vi "Sequence.Compile.vi"(8 "error in (no error)":errorcluster, 11 "State Variables":T10={"Aliases.All"=[], "Aliases.Outputs"=[], "UI.Sequence#ofColumns"=0, "SysDef.Path"=path "", "UI.SequenceRef"=refnum, "UI.StepInformationRef"=refnum, "UI.AbortRef"=refnum, "UI.GraphRef"=refnum, "UI.ViewRef"=refnum, "UI.IterationsRef"=refnum, "UI.IterationInformationRef"=refnum, "INI.Settings"={"Build Location"=path "C:/Simple Sequence Editor/SequenceRepo", "LoggingLocation"=path ""}}) -> (0 "error out":errorcluster, 1 "Warnings":string[](array[string]), 2 "CompiledSettings":T1)   [LabVIEW 2013, in "Simple Sequence Tools - Editor.lvlib"]
uses:
  Simple Sequence Tools - Editor.lvlib
  Types/StateVariables.ctl
  Shared/Types/ChannelProperties.ctl
  Shared/Types/INI.Settings
  Types/Compiled.RTSequenceProperties.ctl
  Types/Compiled.StepProperties.ctl
  Types/Compiled.IOStateProperties.ctl
  Types/Compiled.StepElementProperties.ctl
  Shared/Types/StepTypes.ctl
  Types/Compiled.StepCondition.ctl
  Types/OperationTypes.ctl
  Types/Compiled.SequenceChannels.ctl
  Shared/Simple Sequence Tools - Shared.lvlib
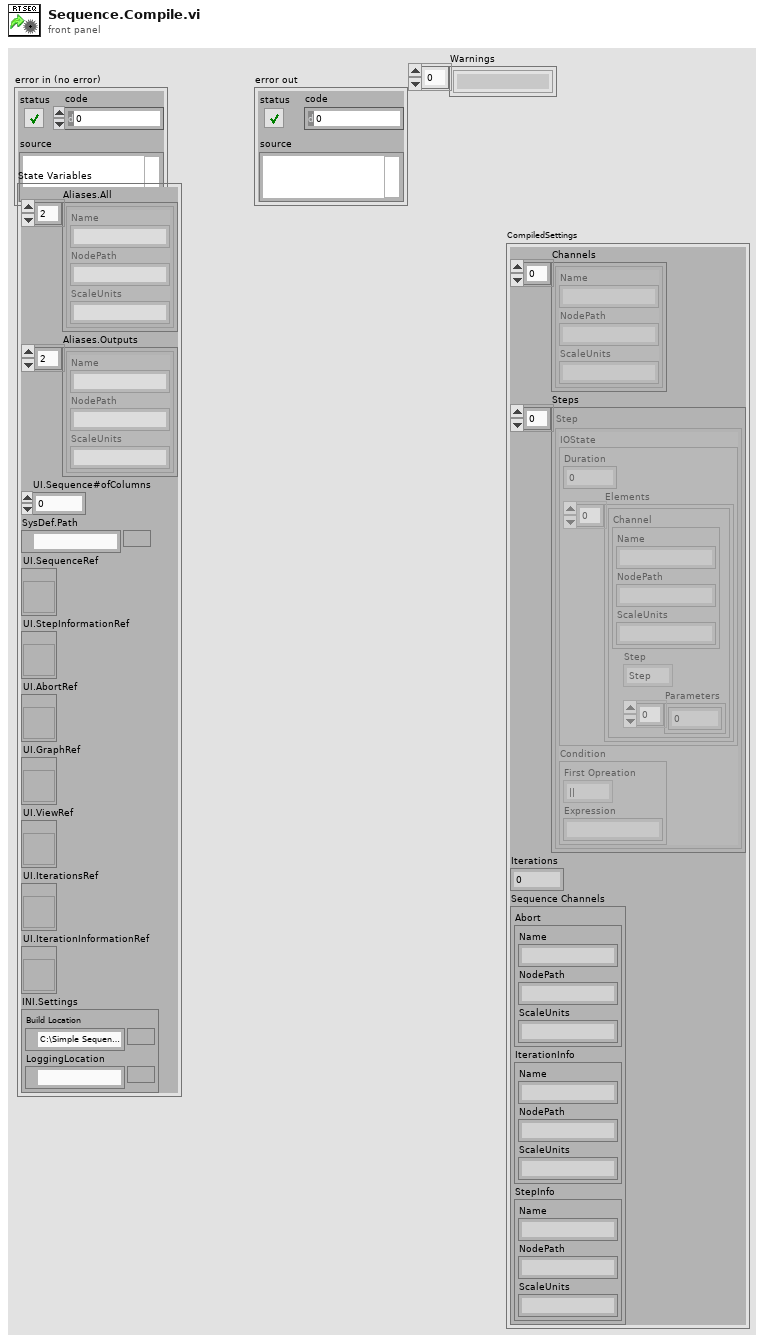
[diagram p1: front panel]
types:
  T1 = typedef "Simple Sequence Tools - Editor.lvlib/Compiled.RTSequenceProperties.ctl" = cluster{"Channels":T2[], "Steps":T3[], "Iterations":u32, "Sequence Channels":T9}
  T2 = typedef "Simple Sequence Tools - Shared.lvlib/ChannelProperties.ctl" = cluster{"Name":string, "NodePath":string, "ScaleUnits":string}
  T3 = typedef "Simple Sequence Tools - Editor.lvlib/Compiled.StepProperties.ctl" = cluster{"IOState":T4, "Condition":T7}
  T4 = typedef "Simple Sequence Tools - Editor.lvlib/Compiled.IOStateProperties.ctl" = cluster{"Duration":dbl, "Elements":T5[]}
  T5 = typedef "Simple Sequence Tools - Editor.lvlib/Compiled.StepElementProperties.ctl" = cluster{"Channel":T2, "Step":T6, "Parameters":dbl[]}
  T6 = typedef "Simple Sequence Tools - Shared.lvlib/StepTypes.ctl" = enum8{"Step", "iStep", "Ramp", "Unchanged", "Unknown"}
  T7 = typedef "Simple Sequence Tools - Editor.lvlib/Compiled.StepCondition.ctl" = cluster{"First Opreation":T8, "Expression":string}
  T8 = typedef "Simple Sequence Tools - Editor.lvlib/OperationTypes.ctl" = enum8{"None", "&&", "||"}
  T9 = typedef "Simple Sequence Tools - Editor.lvlib/Compiled.SequenceChannels.ctl" = cluster{"Abort":T2, "IterationInfo":T2, "StepInfo":T2}
  T10 = typedef "Simple Sequence Tools - Editor.lvlib/StateVariables.ctl" = cluster{"Aliases.All":T2[], "Aliases.Outputs":T2[], "UI.Sequence#ofColumns":i32, "SysDef.Path":path, "UI.SequenceRef":refnum<vi>, "UI.StepInformationRef":refnum<vi>, "UI.AbortRef":refnum<vi>, "UI.GraphRef":refnum<vi>, "UI.ViewRef":refnum<vi>, "UI.IterationsRef":refnum<vi>, "UI.IterationInformationRef":refnum<vi>, "INI.Settings":T11}
  T11 = typedef "Simple Sequence Tools - Shared.lvlib/INI.Settings" = cluster{"Build Location":path, "LoggingLocation":path}
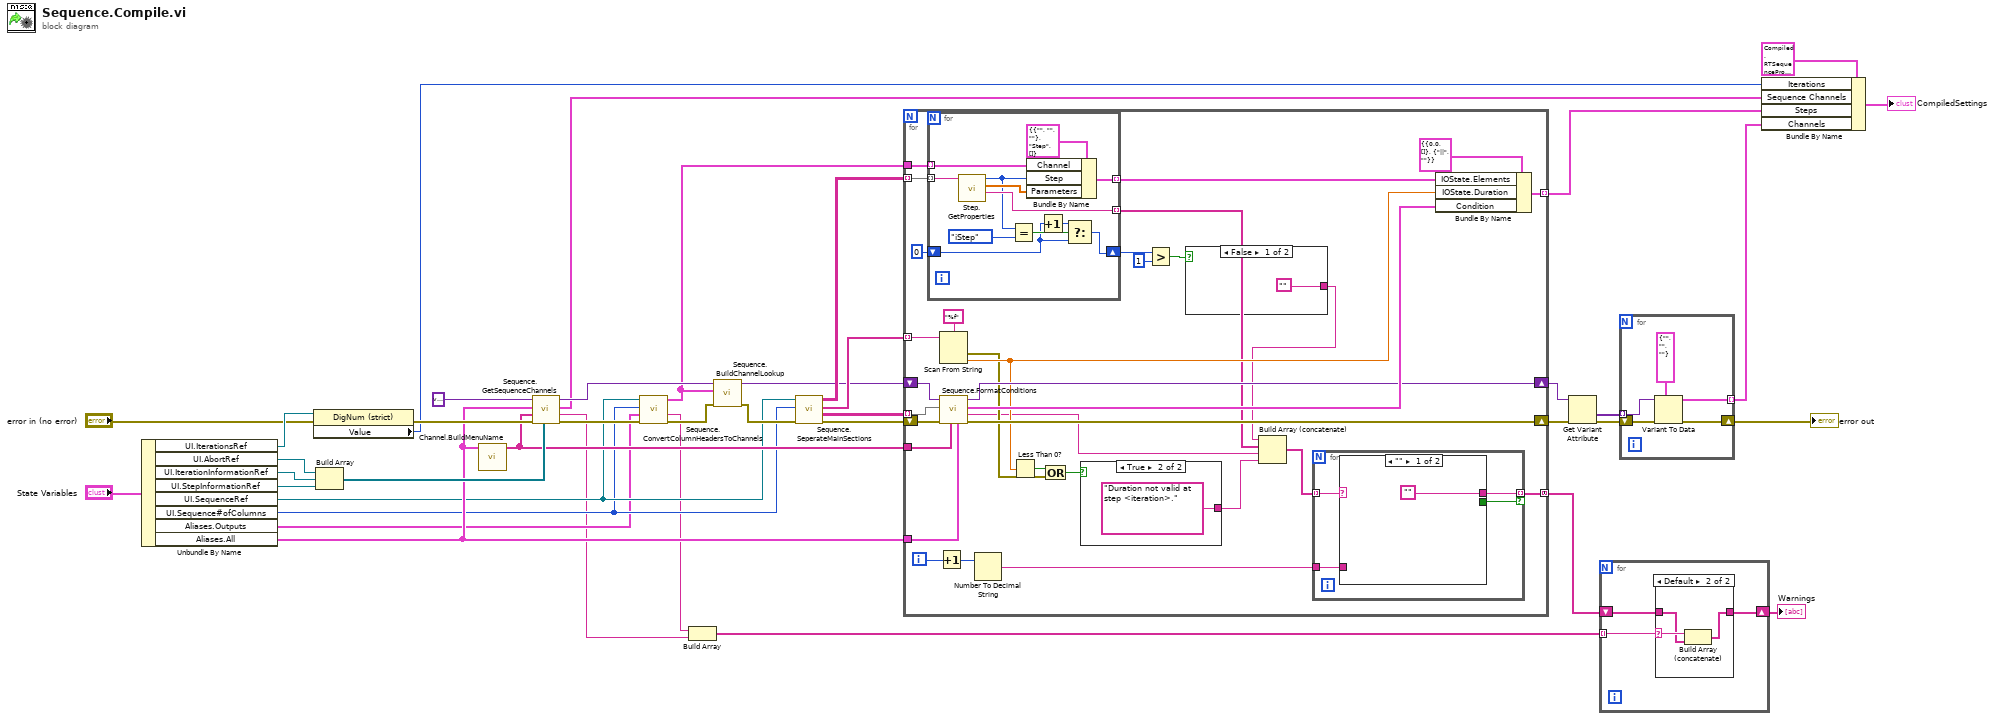
[diagram p0: block diagram]
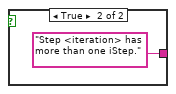
[diagram p3: hidden frame]
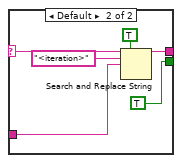
[diagram p4: hidden frame]
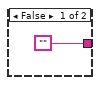
[diagram p5: hidden frame]
diagram:
  n1 = Unbundle By Name("State Variables") -> ("UI.IterationsRef"=w31:refnum<vi>, "UI.AbortRef"=w27:refnum<vi>, "UI.IterationInformationRef"=w26:refnum<vi>, "UI.StepInformationRef"=w25:refnum<vi>, "UI.SequenceRef"=w8:refnum<vi>, "UI.Sequence#ofColumns"=w7:i32, "Aliases.Outputs"=w6:T2[], "Aliases.All"=w20:T2[])
  n2 = property class="DigNum (strict)"(reference=w31, error in="error in (no error)") -> (error out=w24:errorcluster, "Value"=w12:u32)  [unwired: 1 out]
  n3 = Build Array(w27, w26, w25) -> (w23:refnum<vi>[])
  n4 = call "Channel.BuildMenuName.vi"("Aliases"=w20) -> ("Aliases Array"=w19:string[])  [unwired: 10 in]
  n5 = call "Sequence.GetSequenceChannels.vi"("Refs"=w23, "error in (no error)"=w24, "Aliases Array"=w19, "Aliases.All"=w20, "ChannelsLookup"=variant ("variant")) -> ("error out"=w10:errorcluster, "Warnings"=w4:string, "SequenceChannels"=w21:T9, "ChannelsLookup"=w22:variant)  [unwired: 3 in]
  n6 = call "Sequence.ConvertColumnHeadersToChannels.vi"("error in (no error)"=w10, "Aliases.Outputs"=w6, "UI.Sequence#ofColumns"=w7, "UI.SequenceRef"=w8) -> ("error out"=w9:errorcluster, "Warning"=w5:string, "Output Channels"=w16:T2[])  [unwired: 5 in]
  n7 = Build Array(w5, w4) -> (w3:string[])
  n8 = call "Sequence.BuildChannelLookup.vi"("error in (no error)"=w9, "Output Channels"=w16, "ChannelLookup"=w22) -> ("error out"=w18:errorcluster, "ChannelLookup"=w15:variant)  [unwired: 7 in]
  n9 = call "Sequence.SeperateMainSections.vi"("error in (no error)"=w18, "UI.Sequence#ofColumns"=w7, "MulticolumnListbox in"=w8) -> ("error out"=w17:errorcluster, "Conditions"=w36:string[][], "Duration"=w40:string[], "Steps"=w39:string[][])  [unwired: 5 in]
  n10 = for {
    tunnel: w40 -> [w72] mode=indexing
    tunnel: w39 -> [w71] mode=indexing
    tunnel: w16 -> [w70]
    tunnel: [w67] -> w14 mode=indexing
    tunnel: w36 -> [w62] mode=indexing
    tunnel: w19 -> [w63]
    tunnel: w20 -> [w64]
    shift-right: [w66] -> w29
    shift-left: w17 -> [w69]
    shift-right: [w59] -> w28
    shift-left: w15 -> [w61]
    tunnel: [w46] -> w2 mode=concatenating
    i -> [w49]
    n11 = for {
      tunnel: w71 -> [w99] mode=indexing
      tunnel: w70 -> [w97] mode=indexing
      tunnel: [w95] -> w65 mode=indexing
      tunnel: [w94] -> w51 mode=indexing
      shift-right: [w90] -> w44
      shift-left: 0 -> [w89]
      n12 = call "Step.GetProperties.vi"("String in"=w99) -> ("Warning"=w94:string, "Parameters"=w96:dbl[], "Step"=w93:T6)  [unwired: 8 in]
      n13 = Equal?(x=w93, y=StepTypes."iStep") -> (x = y?=w91:bool)
      n14 = Bundle By Name(cluster=T5 {"Channel"={"Name"="", "NodePath"="", "ScaleUnits"=""}, "Step"=enum."Step", "Parameters"=[]}, "Channel"=w97, "Step"=w93, "Parameters"=w96) -> (w95:T5)
      n15 = Increment(x=w89) -> (x+1=w88:i32)
      n16 = Select(t=w88, s=w91, f=w89) -> (s? t:f=w90:i32)
    }
    n17 = Increment(x=w49) -> (x+1=w48:i32)
    n18 = Scan From String(format string="%f", input string=w72) -> (error out=w55:errorcluster, output 1=w57:dbl)  [unwired: 3 in, 2 out]
    n19 = call "Sequence.FormatConditions.vi"("Aliases.All"=w64, "Aliases Array"=w63, "error in (no error)"=w69, "Conditions"=w62, "variant in"=w61) -> ("error out"=w66:errorcluster, "Warning"=w52:string, "Condition"=w60:T7, "variant out"=w59:variant)  [unwired: 3 in]
    n20 = Number To Decimal String(number=w48) -> (decimal integer string=w47:string)  [unwired: 1 in]
    n21 = Less Than 0?(x=w57) -> (x < 0?=w56:bool)
    n22 = Compound Arithmetic op=OR(w56, w55) -> (w54:bool)
    n23 = case shown="True" w54 {
      tunnel: ["" "Duration not valid at step <iteration>."] -> w53
      frame False {
      }
      frame True {
      }
    }
    n24 = Greater?(x=w44, y=1) -> (0:w42:bool)
    n25 = case shown="False" w42 {
      tunnel: ["" "Step <iteration> has more than one iStep."] -> w41
      frame False {
      }
      frame True {
      }
    }
    n26 = Build Array (concatenate)(w41, w51, w52, w53) -> (w50:string[])
    n27 = for {
      tunnel: w50 -> [w77] mode=indexing
      tunnel: w47 -> [w78]
      tunnel: [w76] -> w46 mode=indexing if=w75
      n28 = case shown="\"\"" w77 {
        selector: w77 -> [_ w82]
        tunnel: w78 -> [_ w83]
        tunnel: ["" w81] -> w76
        tunnel: [_ TRUE] -> w75
        frame "" {
        }
        frame Default {
          n29 = Search and Replace String(replace all?=TRUE ("replace all? (F)"), input string=w82, search string="<iteration>", replace string=w83) -> (result string=w81:string)  [unwired: 4 in, 3 out]
        }
      }
    }
    n30 = Bundle By Name(cluster=T3 {"IOState"={"Duration"=0.0, "Elements"=[]}, "Condition"={"First Opreation"=enum."||", "Expression"=""}} ("Step"), "IOState.Elements"=w65, "IOState.Duration"=w57, "Condition"=w60) -> (w67:T3)
  }
  n31 = Get Variant Attribute(Variant=w28, error in=w29) -> (values=w34:variant[], error out=w33:errorcluster)  [unwired: 2 in, 2 out]
  n32 = for {
    tunnel: w3 -> [w102] mode=indexing
    shift-right: [w100] -> w1
    shift-left: w2 -> [w101]
    n33 = case shown="Default" w102 {
      selector: w102 -> [_ w106]
      tunnel: w101 -> [w103 w105]
      tunnel: [w103 w104] -> w100
      frame "" {
      }
      frame Default {
        n34 = Build Array (concatenate)(w106, w105) -> (w104:string[])
      }
    }
  }
  "Warnings" <- w1
  n35 = for {
    tunnel: w34 -> [w111] mode=indexing
    shift-right: [w109] -> w32
    shift-left: w33 -> [w110]
    tunnel: [w107] -> w13 mode=indexing
    n36 = Variant To Data(error in=w110, type=T2 {"Name"="", "NodePath"="", "ScaleUnits"=""} ("cluster"), Variant=w111) -> (data=w107:T2, error out=w109:errorcluster)
  }
  "error out" <- w32
  n37 = Bundle By Name(cluster=T1 {"Channels"=[], "Steps"=[], "Iterations"=0, "Sequence Channels"={"Abort"={"Name"="", "NodePath"="", "ScaleUnits"=""}, "IterationInfo"={"Name"="", "NodePath"="", "ScaleUnits"=""}, "StepInfo"={"Name"="", "NodePath"="", "ScaleUnits"=""}}}, "Iterations"=w12, "Sequence Channels"=w21, "Steps"=w14, "Channels"=w13) -> (→"CompiledSettings":T1)
